vi "Read Reference Power Level.vi"(8 "error in (no error)":errorcluster, 10 "Reference Levels (0)":dbl, 11 "VISA resource name":refnum<visa-resource-name>) -> (0 "error out":errorcluster, 2 "Reference Power Level":dbl, 3 "VISA resource name out":refnum<visa-resource-name>)   [LabVIEW 2018, in "Agilent U2000 Series.lvlib"]
doc: "Finds the reference power level. This provides the reference power level to calculate the pulse parameters.\n\nNote:\nIn case of U2040 X-Series, it is applicable for U2042XA/U2044XA/U2049XA only."
uses:
  Agilent U2000 Series.lvlib
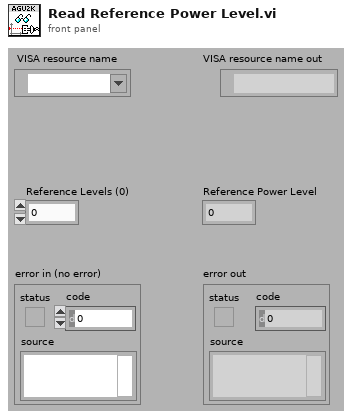
[diagram p1: front panel]
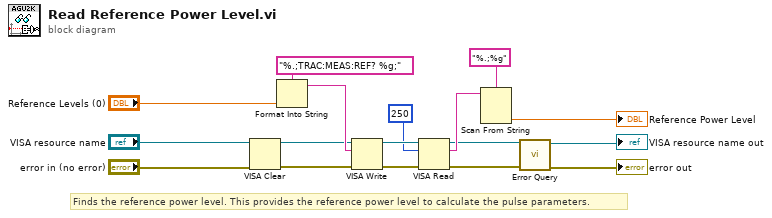
[diagram p0: block diagram]
diagram:
  # "Finds the reference power level. This provides the reference power level to calculate the pulse parameters."
  n1 = VISA Clear(VISA resource name="VISA resource name", error in (no error)="error in (no error)") -> (VISA resource name out=w14:refnum<visa-resource-name>, error out=w13:errorcluster)
  n2 = Format Into String(format string="%.;TRAC:MEAS:REF? %g;", "Reference Levels (0)") -> (resulting string=w15:string)  [unwired: 2 in, 1 out]
  n3 = VISA Write(VISA resource name=w14, write buffer=w15, error in (no error)=w13) -> (VISA resource name out=w9:refnum<visa-resource-name>, error out=w8:errorcluster)  [unwired: 1 out]
  n4 = VISA Read(VISA resource name=w9, byte count=u32 250, error in (no error)=w8) -> (VISA resource name out=w4:refnum<visa-resource-name>, read buffer=w11:string, error out=w3:errorcluster)  [unwired: 1 out]
  n5 = Scan From String(format string="%.;%g", input string=w11) -> (output 1=→"Reference Power Level":dbl)  [unwired: 2 in, 4 out]
  n6 = call "Error Query.vi"("error in (no error)"=w3, "VISA resource name"=w4) -> ("error out"=→"error out":errorcluster, "VISA resource name out"=→"VISA resource name out":refnum<visa-resource-name>)  [unwired: 8 out]
